vi "TIO Data Stream Constant.vi"() -> (0 "TIO State":T1={"Awaiting REP"=FALSE, "REQ ID"=500, "dstreams in"=[], "pstreams"=[], "timebases"=[]})   [LabVIEW 2017]
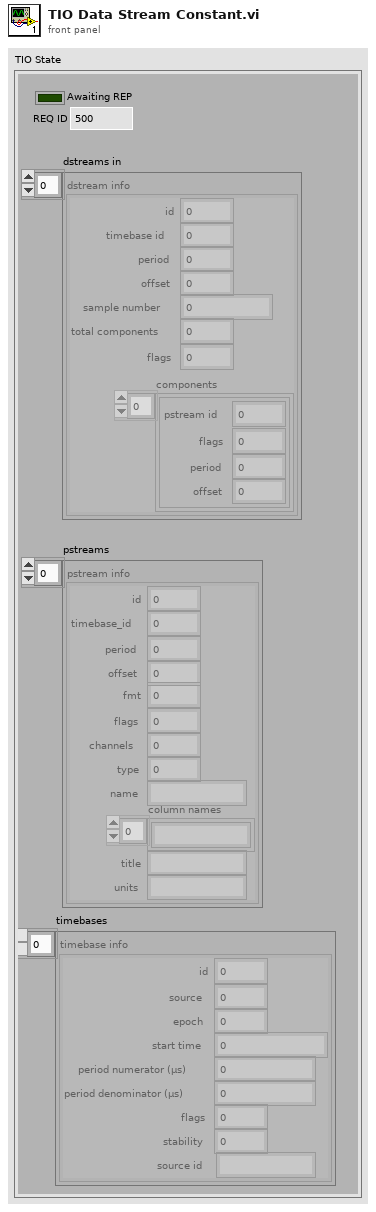
[diagram p1: front panel]
types:
  T1 = cluster{"Awaiting REP":bool, "REQ ID":u32, "dstreams in":cluster{"id":u16, "timebase id":u16, "period":u32, "offset":u32, "sample number":u64, "total components":u16, "flags":u16, "components":cluster{"pstream id":u16, "flags":u16, "period":u32, "offset":u32}[]}[], "pstreams":cluster{"id":u16, "timebase_id":u16, "period":u32, "offset":u32, "fmt":i32, "flags":u16, "channels":u16, "type":u8, "name":string, "column names":string[], "title":string, "units":string}[], "timebases":cluster{"id":u16, "source":u8, "epoch":u8, "start time":u64, "period numerator (µs)":u32, "period denominator (µs)":u32, "flags":u32, "stability":sgl, "source id":string}[]}
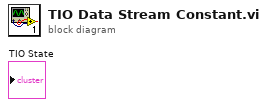
[diagram p0: block diagram]
diagram:
